vi "Error Stop.vi"(8 "error in":errorcluster, 11 "user event":refnum<user-event>) -> (0 "error out":errorcluster)   [LabVIEW 2021]
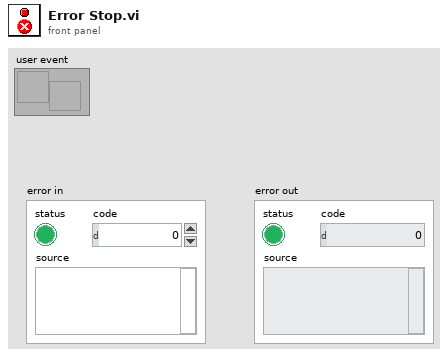
[diagram p1: front panel]
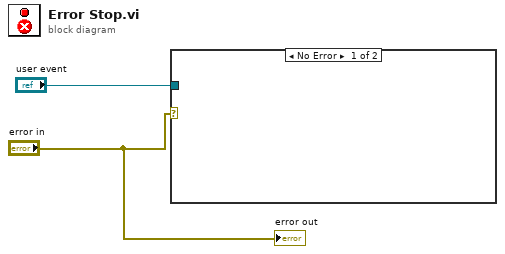
[diagram p0: block diagram]
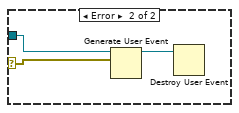
[diagram p2: hidden frame]
diagram:
  n1 = case shown="No Error" "error in" {
    selector: "error in" -> [_ w4]
    tunnel: "user event" -> [_ w5]
    frame No Error {
    }
    frame Error {
      n2 = Generate User Event(user event=w5, event data cluster=w4) -> (user event out=w3:refnum<user-event>)  [unwired: 2 in, 1 out]
      n3 = Destroy User Event(user event=w3) -> ()  [unwired: 1 in, 1 out]
    }
  }
  "error out" <- "error in"
